vi "macro_PIDAutoTune.vi"   [LabVIEW 2019, in "Trajectory_Library.lvlib"]
uses:
  Trajectory_Library.lvlib
types:
  T1 = enum16{"Ziegler Nicols - Fast", "Ziegler Nicols - Normal", "Ziegler Nicols - Slow", "CHR regulator - 0% overshoot", "CHR regulator - 20% overshoot", "CHR servo - 0 % overshoot", "CHR servo - 20% overshoot"}
  T2 = cluster{"Controller Constant Type":enum16{"Ziegler Nicols - Fast", "Ziegler Nicols - Normal", "Ziegler Nicols - Slow", "CHR regulator - 0% overshoot", "CHR regulator - 20% overshoot", "CHR servo - 0 % overshoot", "CHR servo - 20% overshoot"}, "Type of Controller":enum16{"P", "PI", "PID"}, "CO Offset":dbl, "Kn":dbl, "Tuning Tolerance":dbl, "Plant Tolerance":dbl, "Newest Avg Time ":i32, "Long Ave Time":i32}
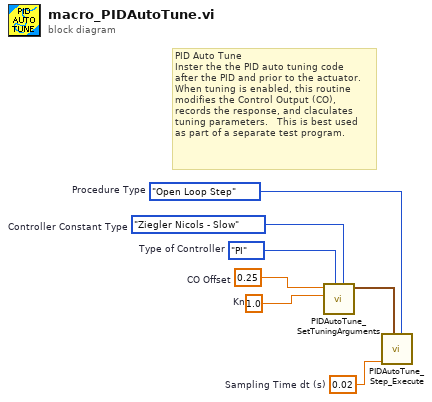
[diagram p0: block diagram]
diagram:
  w1 = 0.02  # Sampling Time dt (s)
  w2 = 1.0  # Kn
  w3 = 0.25  # CO Offset
  w4 = enum16{"P", "PI", "PID"}."PI"  # Type of Controller
  w5 = T1."Ziegler Nicols - Slow"  # Controller Constant Type
  w6 = enum16{"Open Loop Step", "Closed Loop Step"}."Open Loop Step"  # Procedure Type
  # "PID Auto Tune\nInster the the PID auto tuning code\nafter the PID and prior to the actuator.\nWhen tuning is enabled, this routine\nmodifies the Control Output (CO), \nrecords the response, and claculates\ntuning parameters.   This is best used\nas part of a separate test program."
  n1 = call "PIDAutoTune_SetTuningArguments.vi"("Controller Constant Type"=w5, "Type of Controller"=w4, "Kn"=w2, "CO Offset"=w3) -> ("Configuration Parameters"=w7:T2)  [unwired: 7 in]
  n2 = call "PIDAutoTune_Step_Execute.vi"("Procedure Type"=w6, "Configuration Parameters"=w7, "Sampling Time dt (s)"=w1) -> ()  [unwired: 3 in, 6 out]
